vi "_Raise Server Certificate Error Detected.vi"(4 "WebView2.lvlib:WebView2 Control.lvclass":refnum<class "WebView2 Control.lvclass">, 5 "Event Data":cluster{"sender":refnum<k24>, "e":refnum<k24>}, 6 "Control Ref":refnum<k24>, 7 "Event Common Data":T1) -> ()   [LabVIEW 2025, in "WebView2.lvlib" / "WebView2 Control.lvclass"]
uses:
  WebView2 Control.lvclass
  WebView2 Control.lvclass/WebView2 Control.ctl
  E:/Labview/LV 2023/PPL/PPL Builder/Libs/LV-WebView2/Source/Libs/Microsoft.Web.WebView2.Core.dll
  Libs/Microsoft.Web.WebView2.Core.dll
  Server Certificate Error Detected Event Data.ctl
  WebView2 Event Filter Interface/WebView2 Event Filter Interface.lvclass
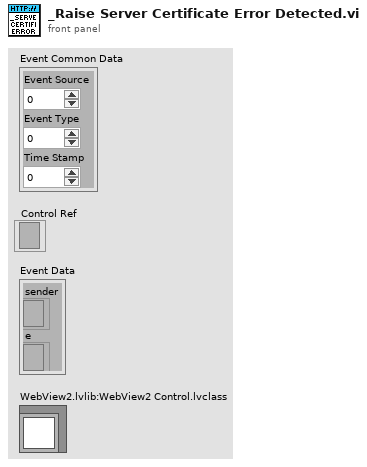
[diagram p1: front panel]
types:
  T1 = cluster{"Event Source":i32, "Event Type":u32, "Time Stamp":u32}
  T2 = typedef "WebView2.lvlib/WebView2 Control.lvclass/Server Certificate Error Detected Event Data.ctl" = cluster{"ErrorStatus":i32, "RequestUri":string, "ServerCertificate":refnum<k24>}
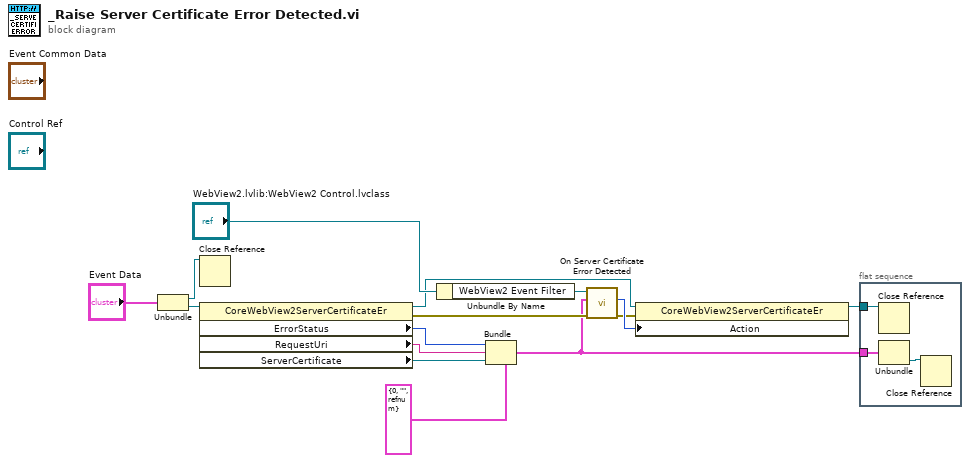
[diagram p0: block diagram]
diagram:
  n1 = Unbundle("Event Data") -> ("sender"=w14:refnum<k24>, "e"=w13:refnum<k24>)
  n2 = Close Reference(reference=w14) -> ()  [unwired: 1 in, 1 out]
  n3 = property class="CoreWebView2ServerCertificateEr"(reference=w13) -> (reference out=w5:refnum<k24>, error out=w6:errorcluster, "ErrorStatus"=w12:i32, "RequestUri"=w11:string, "ServerCertificate"=w10:refnum<k24>)  [unwired: 1 in]
  n4 = Unbundle By Name("WebView2.lvlib:WebView2 Control.lvclass") -> ("WebView2 Event Filter"=w7:refnum<class "WebView2 Event Filter Interface.lvclass">)
  n5 = Bundle(cluster=T2 {"ErrorStatus"=0, "RequestUri"="", "ServerCertificate"=refnum}, "ErrorStatus"=w12, "RequestUri"=w11, "ServerCertificate"=w10) -> (w1:T2)
  n6 = call-dynamic "On Server Certificate Error Detected.vi"("error in (no error)"=w6, "Data"=w1, "WebView2 Event Filter Interface in"=w7) -> ("error out"=w3:errorcluster, "Action"=w4:i32)  [unwired: 7 in]
  n7 = property class="CoreWebView2ServerCertificateEr"(reference=w5, error in=w3, "Action"=w4) -> (reference out=w2:refnum<k24>)  [unwired: 1 out]
  n8 = flat-sequence {
    tunnel: w2 -> [w18]
    tunnel: w1 -> [w17]
    frame #0 {
      n9 = Close Reference(reference=w18) -> ()  [unwired: 1 in, 1 out]
      n10 = Unbundle(w17) -> ("ServerCertificate"=w16:refnum<k24>)  [unwired: 2 out]
      n11 = Close Reference(reference=w16) -> ()  [unwired: 1 in, 1 out]
    }
  }
